vi "Write RobotRef.vi"(8 "error in (no error)":errorcluster, 10 "Robot":refnum<class "Robot.lvclass">, 11 "Role in":refnum<class "Role.lvclass">) -> (0 "error out":errorcluster, 3 "Role out":refnum<class "Role.lvclass">)   [LabVIEW 2023, in "Role.lvclass"]
uses:
  Role.lvclass
  Robot_class/Robot.lvclass
  Role.lvclass/Role.ctl
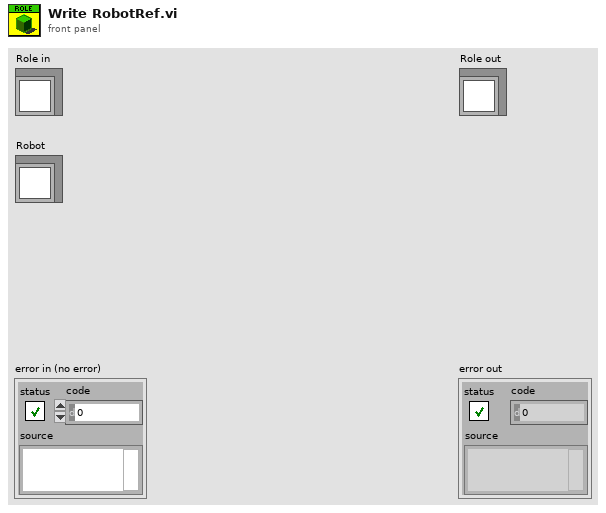
[diagram p1: front panel]
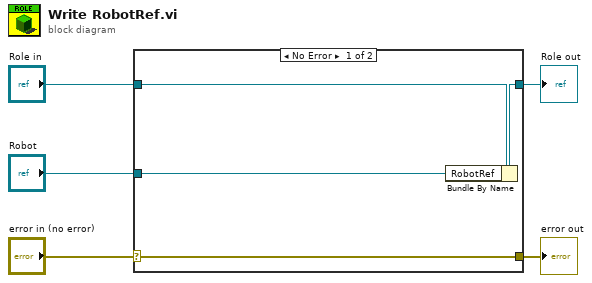
[diagram p0: block diagram]
diagram:
  n1 = case shown="No Error" "error in (no error)" {
    selector: "error in (no error)" -> [w9 w10]
    tunnel: [w9 w10] -> w4
    tunnel: [w7 w11] -> w2
    tunnel: "Role in" -> [w8 w11]
    tunnel: "Robot" -> [w6 _]
    frame No Error {
      n2 = Bundle By Name(cluster=w8, "RobotRef"=w6) -> (w7:refnum<class "Role.lvclass">)
    }
    frame Error {
    }
  }
  "error out" <- w4
  "Role out" <- w2
